vi "GetEventForceActuatorInfoField.vi"(10 "Event Data":string, 11 "Cluster in":refnum<vi>) -> (3 "Array":string[](array[string]))   [LabVIEW 2016]
uses:
  SALLV_m1m3/DataTypes/logevent_ForceActuatorInfo.ctl
  SALLV_m1m3/SALLV_m1m3.lvlib
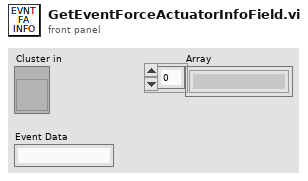
[diagram p1: front panel]
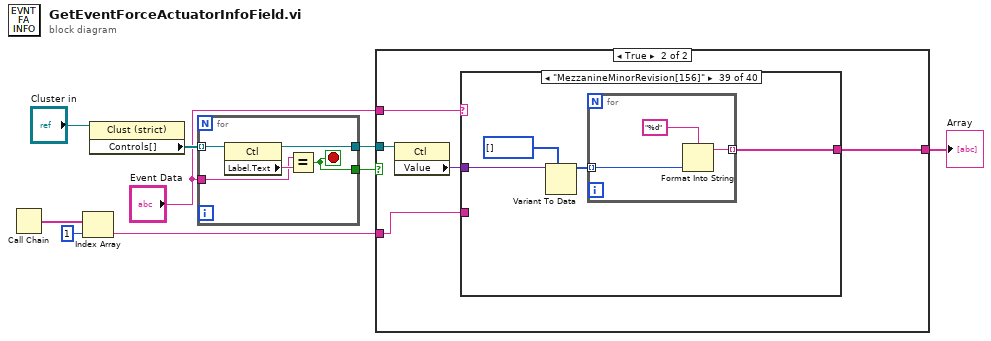
[diagram p0: block diagram]
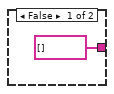
[diagram p2: hidden frame]
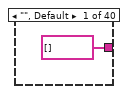
[diagram p3: hidden frame]
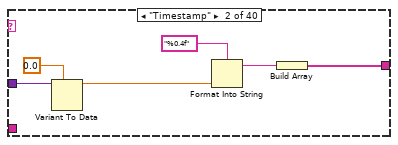
[diagram p4: hidden frame]
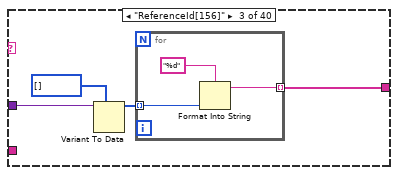
[diagram p5: hidden frame]
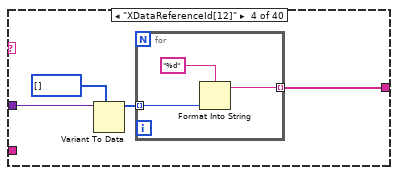
[diagram p6: hidden frame]
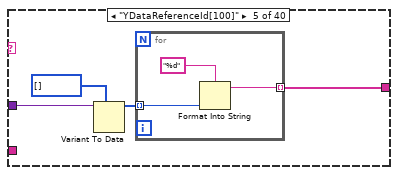
[diagram p7: hidden frame]
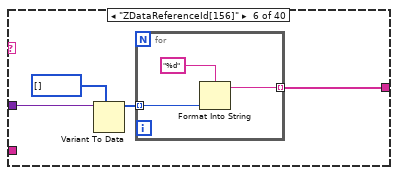
[diagram p8: hidden frame]
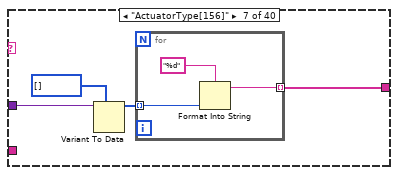
[diagram p9: hidden frame]
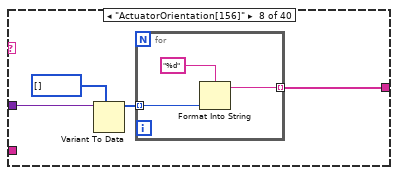
[diagram p10: hidden frame]
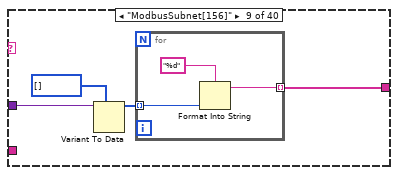
[diagram p11: hidden frame]
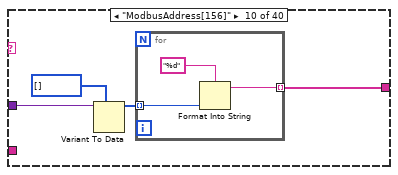
[diagram p12: hidden frame]
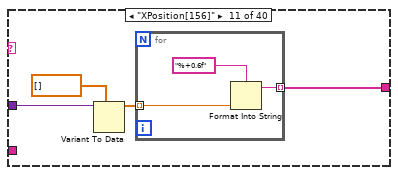
[diagram p13: hidden frame]
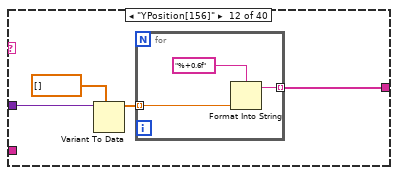
[diagram p14: hidden frame]
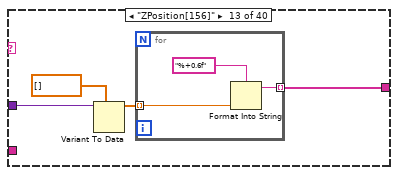
[diagram p15: hidden frame]
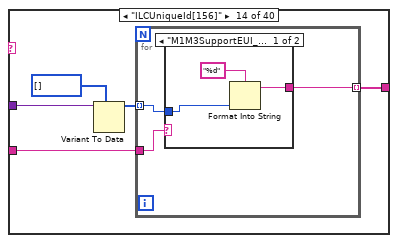
[diagram p16: hidden frame]
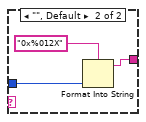
[diagram p17: hidden frame]
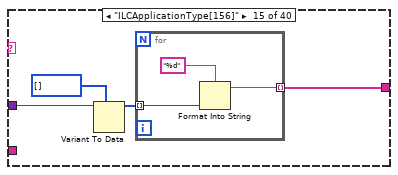
[diagram p18: hidden frame]
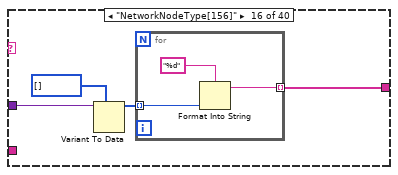
[diagram p19: hidden frame]
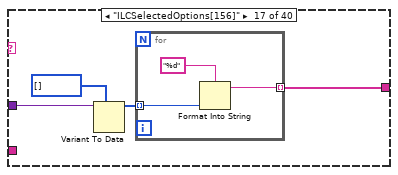
[diagram p20: hidden frame]
diagram:
  n1 = Call Chain() -> (call chain=w3:string[])
  n2 = Index Array(array=w3, index=1) -> (element=w1:string)
  n3 = property on="Property Node" class="Clust (strict)"(reference="Cluster in") -> ("Controls[]"=w9:refnum<vi>[])  [unwired: 1 in, 2 out]
  n4 = for {
    tunnel: w9 -> [w14] mode=indexing
    tunnel: [w13] -> w4
    tunnel: "Event Data" -> [w11]
    tunnel: [w10] -> w5
    stop <- w10 stop-if-true
    n5 = property on="Property Node" class="Ctl"(reference=w14) -> (reference out=w13:refnum<vi>, "Label.Text"=w12:string)  [unwired: 1 in, 1 out]
    n6 = Equal?(x=w11, y=w12) -> (x = y?=w10:bool)
  }
  n7 = case shown="True" w5 {
    tunnel: "Event Data" -> [_ w20]
    tunnel: w4 -> [_ w19]
    tunnel: [string[] [] w17] -> w7
    tunnel: w1 -> [_ w16]
    frame False {
    }
    frame True {
      n8 = property on="Property Node" class="Ctl"(reference=w19) -> ("Value"=w18:variant)  [unwired: 1 in, 2 out]
      n9 = case shown="\"MezzanineMinorRevision[156]\"" w20 {
        tunnel: [string[] [] w25 w28 w35 w42 w49 w56 w63 w70 w77 w84 w91 w98 w106 w119 w126 w133 w140 w147 w154 w161 w168 w175 w182 w189 w196 w203 w210 w217 w224 w231 w238 w245 w252 w259 w267 w280 w287 w294 w304] -> w17
        tunnel: w18 -> [_ w23 w31 w38 w45 w52 w59 w66 w73 w80 w87 w94 w101 w109 w122 w129 w136 w143 w150 w157 w164 w171 w178 w185 w192 w199 w206 w213 w220 w227 w234 w241 w248 w255 w262 w270 w283 w290 w297 w302]
        tunnel: w16 -> [_ _ _ _ _ _ _ _ _ _ _ _ _ w105 _ _ _ _ _ _ _ _ _ _ _ _ _ _ _ _ _ _ _ _ _ w266 _ _ _ _]
        frame "", Default {
        }
        frame "Timestamp" {
          n10 = Variant To Data(type=0.0, Variant=w23) -> (data=w24:dbl)  [unwired: 1 in, 1 out]
          n11 = Format Into String(format string="%0.4f", w24) -> (resulting string=w26:string)  [unwired: 2 in, 1 out]
          n12 = Build Array(w26) -> (w25:string[])
        }
        frame "ReferenceId[156]" {
          n13 = Variant To Data(type=i16[] [], Variant=w31) -> (data=w29:i16[])  [unwired: 1 in, 1 out]
          n14 = for {
            tunnel: w29 -> [w33] mode=indexing
            tunnel: [w32] -> w28 mode=indexing
            n15 = Format Into String(format string="%d", w33) -> (resulting string=w32:string)  [unwired: 2 in, 1 out]
          }
        }
        frame "XDataReferenceId[12]" {
          n16 = Variant To Data(type=i32[] [], Variant=w38) -> (data=w36:i32[])  [unwired: 1 in, 1 out]
          n17 = for {
            tunnel: w36 -> [w40] mode=indexing
            tunnel: [w39] -> w35 mode=indexing
            n18 = Format Into String(format string="%d", w40) -> (resulting string=w39:string)  [unwired: 2 in, 1 out]
          }
        }
        frame "YDataReferenceId[100]" {
          n19 = Variant To Data(type=i32[] [], Variant=w45) -> (data=w43:i32[])  [unwired: 1 in, 1 out]
          n20 = for {
            tunnel: w43 -> [w47] mode=indexing
            tunnel: [w46] -> w42 mode=indexing
            n21 = Format Into String(format string="%d", w47) -> (resulting string=w46:string)  [unwired: 2 in, 1 out]
          }
        }
        frame "ZDataReferenceId[156]" {
          n22 = Variant To Data(type=i32[] [], Variant=w52) -> (data=w50:i32[])  [unwired: 1 in, 1 out]
          n23 = for {
            tunnel: w50 -> [w54] mode=indexing
            tunnel: [w53] -> w49 mode=indexing
            n24 = Format Into String(format string="%d", w54) -> (resulting string=w53:string)  [unwired: 2 in, 1 out]
          }
        }
        frame "ActuatorType[156]" {
          n25 = Variant To Data(type=i32[] [], Variant=w59) -> (data=w57:i32[])  [unwired: 1 in, 1 out]
          n26 = for {
            tunnel: w57 -> [w61] mode=indexing
            tunnel: [w60] -> w56 mode=indexing
            n27 = Format Into String(format string="%d", w61) -> (resulting string=w60:string)  [unwired: 2 in, 1 out]
          }
        }
        frame "ActuatorOrientation[156]" {
          n28 = Variant To Data(type=i32[] [], Variant=w66) -> (data=w64:i32[])  [unwired: 1 in, 1 out]
          n29 = for {
            tunnel: w64 -> [w68] mode=indexing
            tunnel: [w67] -> w63 mode=indexing
            n30 = Format Into String(format string="%d", w68) -> (resulting string=w67:string)  [unwired: 2 in, 1 out]
          }
        }
        frame "ModbusSubnet[156]" {
          n31 = Variant To Data(type=i16[] [], Variant=w73) -> (data=w71:i16[])  [unwired: 1 in, 1 out]
          n32 = for {
            tunnel: w71 -> [w75] mode=indexing
            tunnel: [w74] -> w70 mode=indexing
            n33 = Format Into String(format string="%d", w75) -> (resulting string=w74:string)  [unwired: 2 in, 1 out]
          }
        }
        frame "ModbusAddress[156]" {
          n34 = Variant To Data(type=i16[] [], Variant=w80) -> (data=w78:i16[])  [unwired: 1 in, 1 out]
          n35 = for {
            tunnel: w78 -> [w82] mode=indexing
            tunnel: [w81] -> w77 mode=indexing
            n36 = Format Into String(format string="%d", w82) -> (resulting string=w81:string)  [unwired: 2 in, 1 out]
          }
        }
        frame "XPosition[156]" {
          n37 = Variant To Data(type=sgl[] [], Variant=w87) -> (data=w85:sgl[])  [unwired: 1 in, 1 out]
          n38 = for {
            tunnel: w85 -> [w89] mode=indexing
            tunnel: [w88] -> w84 mode=indexing
            n39 = Format Into String(format string="%+0.6f", w89) -> (resulting string=w88:string)  [unwired: 2 in, 1 out]
          }
        }
        frame "YPosition[156]" {
          n40 = Variant To Data(type=sgl[] [], Variant=w94) -> (data=w92:sgl[])  [unwired: 1 in, 1 out]
          n41 = for {
            tunnel: w92 -> [w96] mode=indexing
            tunnel: [w95] -> w91 mode=indexing
            n42 = Format Into String(format string="%+0.6f", w96) -> (resulting string=w95:string)  [unwired: 2 in, 1 out]
          }
        }
        frame "ZPosition[156]" {
          n43 = Variant To Data(type=sgl[] [], Variant=w101) -> (data=w99:sgl[])  [unwired: 1 in, 1 out]
          n44 = for {
            tunnel: w99 -> [w103] mode=indexing
            tunnel: [w102] -> w98 mode=indexing
            n45 = Format Into String(format string="%+0.6f", w103) -> (resulting string=w102:string)  [unwired: 2 in, 1 out]
          }
        }
        frame "ILCUniqueId[156]" {
          n46 = Variant To Data(type=i64[] [], Variant=w109) -> (data=w107:i64[])  [unwired: 1 in, 1 out]
          n47 = for {
            tunnel: w107 -> [w112] mode=indexing
            tunnel: [w111] -> w106 mode=indexing
            tunnel: w105 -> [w110]
            n48 = case shown="\"M1M3SupportEUI_Views.lvlib:FA Graphic View.vi\"" w110 {
              tunnel: [w114 w116] -> w111
              tunnel: w112 -> [w113 w117]
              frame "M1M3SupportEUI_Views.lvlib:FA Graphic View.vi" {
                n49 = Format Into String(format string="%d", w113) -> (resulting string=w114:string)  [unwired: 2 in, 1 out]
              }
              frame "", Default {
                n50 = Format Into String(format string="0x%012X", w117) -> (resulting string=w116:string)  [unwired: 2 in, 1 out]
              }
            }
          }
        }
        frame "ILCApplicationType[156]" {
          n51 = Variant To Data(type=i16[] [], Variant=w122) -> (data=w120:i16[])  [unwired: 1 in, 1 out]
          n52 = for {
            tunnel: w120 -> [w124] mode=indexing
            tunnel: [w123] -> w119 mode=indexing
            n53 = Format Into String(format string="%d", w124) -> (resulting string=w123:string)  [unwired: 2 in, 1 out]
          }
        }
        frame "NetworkNodeType[156]" {
          n54 = Variant To Data(type=i16[] [], Variant=w129) -> (data=w127:i16[])  [unwired: 1 in, 1 out]
          n55 = for {
            tunnel: w127 -> [w131] mode=indexing
            tunnel: [w130] -> w126 mode=indexing
            n56 = Format Into String(format string="%d", w131) -> (resulting string=w130:string)  [unwired: 2 in, 1 out]
          }
        }
        frame "ILCSelectedOptions[156]" {
          n57 = Variant To Data(type=i16[] [], Variant=w136) -> (data=w134:i16[])  [unwired: 1 in, 1 out]
          n58 = for {
            tunnel: w134 -> [w138] mode=indexing
            tunnel: [w137] -> w133 mode=indexing
            n59 = Format Into String(format string="%d", w138) -> (resulting string=w137:string)  [unwired: 2 in, 1 out]
          }
        }
        frame "NetworkNodeOptions[156]" {
          n60 = Variant To Data(type=i16[] [], Variant=w143) -> (data=w141:i16[])  [unwired: 1 in, 1 out]
          n61 = for {
            tunnel: w141 -> [w145] mode=indexing
            tunnel: [w144] -> w140 mode=indexing
            n62 = Format Into String(format string="%d", w145) -> (resulting string=w144:string)  [unwired: 2 in, 1 out]
          }
        }
        frame "MajorRevision[156]" {
          n63 = Variant To Data(type=i16[] [], Variant=w150) -> (data=w148:i16[])  [unwired: 1 in, 1 out]
          n64 = for {
            tunnel: w148 -> [w152] mode=indexing
            tunnel: [w151] -> w147 mode=indexing
            n65 = Format Into String(format string="%d", w152) -> (resulting string=w151:string)  [unwired: 2 in, 1 out]
          }
        }
        frame "MinorRevision[156]" {
          n66 = Variant To Data(type=i16[] [], Variant=w157) -> (data=w155:i16[])  [unwired: 1 in, 1 out]
          n67 = for {
            tunnel: w155 -> [w159] mode=indexing
            tunnel: [w158] -> w154 mode=indexing
            n68 = Format Into String(format string="%d", w159) -> (resulting string=w158:string)  [unwired: 2 in, 1 out]
          }
        }
        frame "ADCScanRate[156]" {
          n69 = Variant To Data(type=i16[] [], Variant=w164) -> (data=w162:i16[])  [unwired: 1 in, 1 out]
          n70 = for {
            tunnel: w162 -> [w166] mode=indexing
            tunnel: [w165] -> w161 mode=indexing
            n71 = Format Into String(format string="%d", w166) -> (resulting string=w165:string)  [unwired: 2 in, 1 out]
          }
        }
        frame "MainPrimaryCylinderCoefficient[156]" {
          n72 = Variant To Data(type=sgl[] [], Variant=w171) -> (data=w169:sgl[])  [unwired: 1 in, 1 out]
          n73 = for {
            tunnel: w169 -> [w173] mode=indexing
            tunnel: [w172] -> w168 mode=indexing
            n74 = Format Into String(format string="%+0.9f", w173) -> (resulting string=w172:string)  [unwired: 2 in, 1 out]
          }
        }
        frame "MainSecondaryCylinderCoefficient[156]" {
          n75 = Variant To Data(type=sgl[] [], Variant=w178) -> (data=w176:sgl[])  [unwired: 1 in, 1 out]
          n76 = for {
            tunnel: w176 -> [w180] mode=indexing
            tunnel: [w179] -> w175 mode=indexing
            n77 = Format Into String(format string="%+0.9f", w180) -> (resulting string=w179:string)  [unwired: 2 in, 1 out]
          }
        }
        frame "MainPrimaryCylinderLoadCellOffset[156]" {
          n78 = Variant To Data(type=sgl[] [], Variant=w185) -> (data=w183:sgl[])  [unwired: 1 in, 1 out]
          n79 = for {
            tunnel: w183 -> [w187] mode=indexing
            tunnel: [w186] -> w182 mode=indexing
            n80 = Format Into String(format string="%+0.3f", w187) -> (resulting string=w186:string)  [unwired: 2 in, 1 out]
          }
        }
        frame "MainSecondaryCylinderLoadCellOffset[156]" {
          n81 = Variant To Data(type=sgl[] [], Variant=w192) -> (data=w190:sgl[])  [unwired: 1 in, 1 out]
          n82 = for {
            tunnel: w190 -> [w194] mode=indexing
            tunnel: [w193] -> w189 mode=indexing
            n83 = Format Into String(format string="%+0.3f", w194) -> (resulting string=w193:string)  [unwired: 2 in, 1 out]
          }
        }
        frame "MainPrimaryCylinderLoadCellSensitivity[156]" {
          n84 = Variant To Data(type=sgl[] [], Variant=w199) -> (data=w197:sgl[])  [unwired: 1 in, 1 out]
          n85 = for {
            tunnel: w197 -> [w201] mode=indexing
            tunnel: [w200] -> w196 mode=indexing
            n86 = Format Into String(format string="%+0.3f", w201) -> (resulting string=w200:string)  [unwired: 2 in, 1 out]
          }
        }
        frame "MainSecondaryCylinderLoadCellSensitivity[156]" {
          n87 = Variant To Data(type=sgl[] [], Variant=w206) -> (data=w204:sgl[])  [unwired: 1 in, 1 out]
          n88 = for {
            tunnel: w204 -> [w208] mode=indexing
            tunnel: [w207] -> w203 mode=indexing
            n89 = Format Into String(format string="%+0.3f", w208) -> (resulting string=w207:string)  [unwired: 2 in, 1 out]
          }
        }
        frame "BackupPrimaryCylinderCoefficient[156]" {
          n90 = Variant To Data(type=sgl[] [], Variant=w213) -> (data=w211:sgl[])  [unwired: 1 in, 1 out]
          n91 = for {
            tunnel: w211 -> [w215] mode=indexing
            tunnel: [w214] -> w210 mode=indexing
            n92 = Format Into String(format string="%+0.9f", w215) -> (resulting string=w214:string)  [unwired: 2 in, 1 out]
          }
        }
        frame "BackupSecondaryCylinderCoefficient[156]" {
          n93 = Variant To Data(type=sgl[] [], Variant=w220) -> (data=w218:sgl[])  [unwired: 1 in, 1 out]
          n94 = for {
            tunnel: w218 -> [w222] mode=indexing
            tunnel: [w221] -> w217 mode=indexing
            n95 = Format Into String(format string="%+0.9f", w222) -> (resulting string=w221:string)  [unwired: 2 in, 1 out]
          }
        }
        frame "BackupPrimaryCylinderLoadCellOffset[156]" {
          n96 = Variant To Data(type=sgl[] [], Variant=w227) -> (data=w225:sgl[])  [unwired: 1 in, 1 out]
          n97 = for {
            tunnel: w225 -> [w229] mode=indexing
            tunnel: [w228] -> w224 mode=indexing
            n98 = Format Into String(format string="%+0.3f", w229) -> (resulting string=w228:string)  [unwired: 2 in, 1 out]
          }
        }
        frame "BackupSecondaryCylinderLoadCellOffset[156]" {
          n99 = Variant To Data(type=sgl[] [], Variant=w234) -> (data=w232:sgl[])  [unwired: 1 in, 1 out]
          n100 = for {
            tunnel: w232 -> [w236] mode=indexing
            tunnel: [w235] -> w231 mode=indexing
            n101 = Format Into String(format string="%+0.3f", w236) -> (resulting string=w235:string)  [unwired: 2 in, 1 out]
          }
        }
        frame "BackupPrimaryCylinderLoadCellSensitivity[156]" {
          n102 = Variant To Data(type=sgl[] [], Variant=w241) -> (data=w239:sgl[])  [unwired: 1 in, 1 out]
          n103 = for {
            tunnel: w239 -> [w243] mode=indexing
            tunnel: [w242] -> w238 mode=indexing
            n104 = Format Into String(format string="%+0.3f", w243) -> (resulting string=w242:string)  [unwired: 2 in, 1 out]
          }
        }
        frame "BackupSecondaryCylinderLoadCellSensitivity[156]" {
          n105 = Variant To Data(type=sgl[] [], Variant=w248) -> (data=w246:sgl[])  [unwired: 1 in, 1 out]
          n106 = for {
            tunnel: w246 -> [w250] mode=indexing
            tunnel: [w249] -> w245 mode=indexing
            n107 = Format Into String(format string="%+0.3f", w250) -> (resulting string=w249:string)  [unwired: 2 in, 1 out]
          }
        }
        frame "MezzaninePrimaryCylinderGain[156]" {
          n108 = Variant To Data(type=sgl[] [], Variant=w255) -> (data=w253:sgl[])  [unwired: 1 in, 1 out]
          n109 = for {
            tunnel: w253 -> [w257] mode=indexing
            tunnel: [w256] -> w252 mode=indexing
            n110 = Format Into String(format string="%+0.3f", w257) -> (resulting string=w256:string)  [unwired: 2 in, 1 out]
          }
        }
        frame "MezzanineSecondaryCylinderGain[156]" {
          n111 = Variant To Data(type=sgl[] [], Variant=w262) -> (data=w260:sgl[])  [unwired: 1 in, 1 out]
          n112 = for {
            tunnel: w260 -> [w264] mode=indexing
            tunnel: [w263] -> w259 mode=indexing
            n113 = Format Into String(format string="%+0.3f", w264) -> (resulting string=w263:string)  [unwired: 2 in, 1 out]
          }
        }
        frame "MezzanineUniqueId[156]" {
          n114 = Variant To Data(type=i64[] [], Variant=w270) -> (data=w268:i64[])  [unwired: 1 in, 1 out]
          n115 = for {
            tunnel: w268 -> [w273] mode=indexing
            tunnel: [w272] -> w267 mode=indexing
            tunnel: w266 -> [w271]
            n116 = case shown="\"M1M3SupportEUI_Views.lvlib:FA Graphic View.vi\"" w271 {
              tunnel: [w275 w277] -> w272
              tunnel: w273 -> [w274 w278]
              frame "M1M3SupportEUI_Views.lvlib:FA Graphic View.vi" {
                n117 = Format Into String(format string="%d", w274) -> (resulting string=w275:string)  [unwired: 2 in, 1 out]
              }
              frame "", Default {
                n118 = Format Into String(format string="0x%012X", w278) -> (resulting string=w277:string)  [unwired: 2 in, 1 out]
              }
            }
          }
        }
        frame "MezzanineFirmwareType[156]" {
          n119 = Variant To Data(type=i16[] [], Variant=w283) -> (data=w281:i16[])  [unwired: 1 in, 1 out]
          n120 = for {
            tunnel: w281 -> [w285] mode=indexing
            tunnel: [w284] -> w280 mode=indexing
            n121 = Format Into String(format string="%d", w285) -> (resulting string=w284:string)  [unwired: 2 in, 1 out]
          }
        }
        frame "MezzanineMajorRevision[156]" {
          n122 = Variant To Data(type=i16[] [], Variant=w290) -> (data=w288:i16[])  [unwired: 1 in, 1 out]
          n123 = for {
            tunnel: w288 -> [w292] mode=indexing
            tunnel: [w291] -> w287 mode=indexing
            n124 = Format Into String(format string="%d", w292) -> (resulting string=w291:string)  [unwired: 2 in, 1 out]
          }
        }
        frame "MezzanineMinorRevision[156]" {
          n125 = Variant To Data(type=i16[] [], Variant=w297) -> (data=w295:i16[])  [unwired: 1 in, 1 out]
          n126 = for {
            tunnel: w295 -> [w299] mode=indexing
            tunnel: [w298] -> w294 mode=indexing
            n127 = Format Into String(format string="%d", w299) -> (resulting string=w298:string)  [unwired: 2 in, 1 out]
          }
        }
        frame "priority" {
          n128 = Variant To Data(type=0, Variant=w302) -> (data=w303:i32)  [unwired: 1 in, 1 out]
          n129 = Format Into String(format string="%d", w303) -> (resulting string=w305:string)  [unwired: 2 in, 1 out]
          n130 = Build Array(w305) -> (w304:string[])
        }
      }
    }
  }
  "Array" <- w7
